vi "Configure Timer Interval Error Filter Shape.vi"(8 "error in (no error)":errorcluster, 10 "Filter Shape (0: RECT)":i32(ring) items=["Rectangular", "20 dB Per Decade", "40 dB Per Decade"], 11 "VISA resource name":refnum<visa-resource-name>) -> (0 "error out":errorcluster, 3 "VISA resource name out":refnum<visa-resource-name>)   [LabVIEW 2013, in "Agilent 90000 Series.lvlib"]
doc: "Configures the shape of the TIE filter edge."
uses:
  Agilent 90000 Series.lvlib
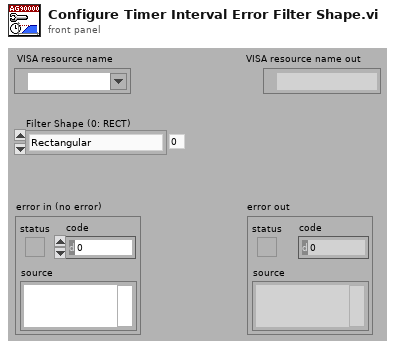
[diagram p1: front panel]
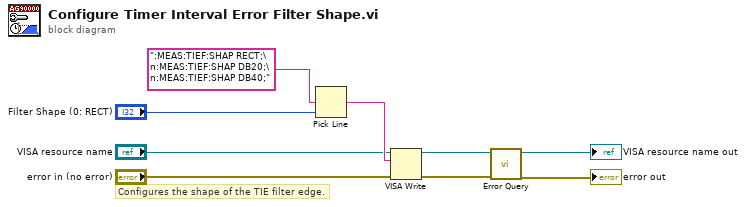
[diagram p0: block diagram]
diagram:
  # "Configures the shape of the TIE filter edge."
  n1 = Pick Line(multi-line string=":MEAS:TIEF:SHAP RECT;\n:MEAS:TIEF:SHAP DB20;\n:MEAS:TIEF:SHAP DB40;", line index="Filter Shape (0: RECT)") -> (output string=w7:string)  [unwired: 1 out]
  n2 = VISA Write(VISA resource name="VISA resource name", write buffer=w7, error in (no error)="error in (no error)") -> (VISA resource name out=w4:refnum<visa-resource-name>, error out=w3:errorcluster)  [unwired: 1 out]
  n3 = call "Error Query.vi"("error in (no error)"=w3, "VISA resource name"=w4) -> ("error out"=→"error out":errorcluster, "VISA resource name out"=→"VISA resource name out":refnum<visa-resource-name>)  [unwired: 8 out]
